vi "connectCommandPublish.vi"(8 "error in (no error)":errorcluster, 11 "MiddlewareSVThisComponent in":refnum<class "MiddlewareSVThisComponent.lvclass">) -> (0 "error out":errorcluster, 3 "MiddlewareSVThisComponent out":refnum<class "MiddlewareSVThisComponent.lvclass">)   [LabVIEW 2015, in "MiddlewareSVThisComponent.lvclass"]
uses:
  MiddlewareSVThisComponent.lvclass
  ComponentTemplateCore/ComponentModel/ComponentModel/Typedefs/CommunicationConfig.ctl
  ComponentTemplateCore/ComponentModel/ComponentModel/Typedefs/SVProcessConfig.ctl
  ComponentTemplateCore/ComponentModel/ComponentModelDT/ConfigurationFileReaderDT/ConfigurationFileReaderDT.lvclass
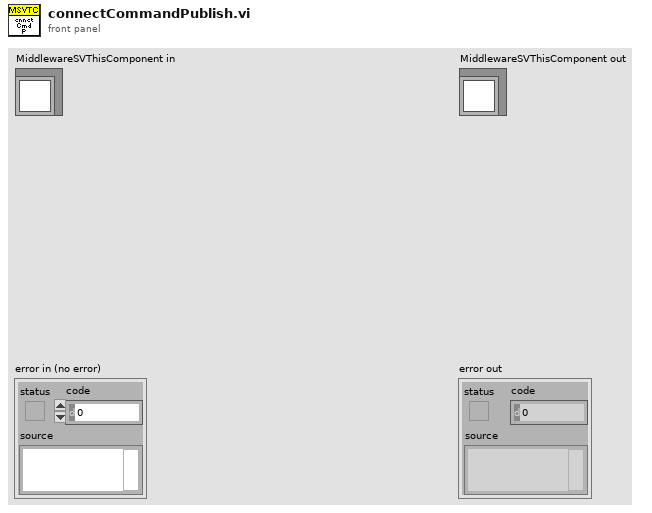
[diagram p1: front panel]
types:
  T1 = typedef "SVProcessConfig.ctl" = cluster{"subDataProcessPrototype":string, "pubDataProcessPrototype":string, "commandProcessPrototype":string, "commandSVName":string}
  T2 = typedef "CommunicationConfig.ctl" = cluster{"hostComputerAddress":string, "ComponentAcronym":string, "InstanceIdentifier":i32}
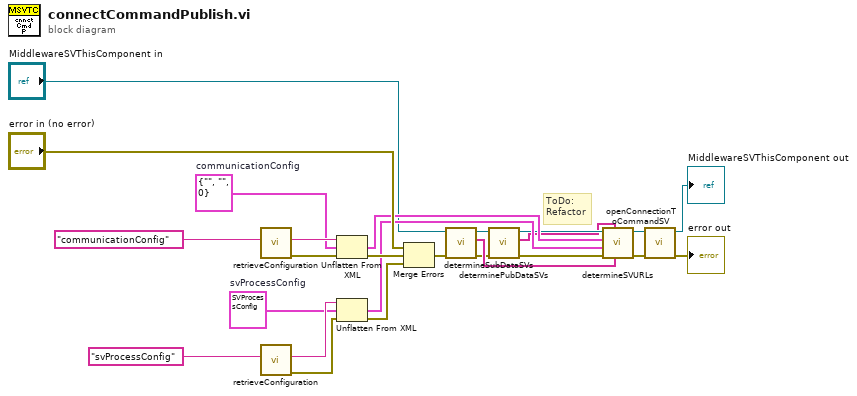
[diagram p0: block diagram]
diagram:
  w18 = T1 {"subDataProcessPrototype"="SubDataSV", "pubDataProcessPrototype"="PubDataSV", "commandProcessPrototype"="CommandSV", "commandSVName"="Command"}  # svProcessConfig
  w22 = T2 {"hostComputerAddress"="", "ComponentAcronym"="", "InstanceIdentifier"=0}  # communicationConfig
  # "ToDo:\nRefactor"
  n1 = call "retrieveConfiguration.vi"("dataName"="communicationConfig") -> ("error out"=w23:errorcluster, "dataValueFromFile"=w24:string)  [unwired: 8 in, 1 out]
  n2 = call "retrieveConfiguration.vi"("dataName"="svProcessConfig") -> ("error out"=w21:errorcluster, "dataValueFromFile"=w20:string)  [unwired: 8 in, 1 out]
  n3 = Unflatten From XML(xml string=w24, type=w22, error in (no error)=w23) -> (value=w9:T2, error out=w17:errorcluster)
  n4 = Unflatten From XML(xml string=w20, type=w18, error in (no error)=w21) -> (value=w10:T1, error out=w16:errorcluster)
  n5 = Merge Errors("error in (no error)", w17, w16) -> (w7:errorcluster)
  n6 = call "determineSubDataSVs.vi"("error in (no error)"=w7, "MiddlewareSVThisComponent in"="MiddlewareSVThisComponent in") -> ("error out"=w2:errorcluster, "svNames"=w6:string[], "MiddlewareSVThisComponent out"=w5:refnum<class "MiddlewareSVThisComponent.lvclass">)  [unwired: 7 in]
  n7 = call "determinePubDataSVs.vi"("error in (no error)"=w2, "MiddlewareSVThisComponent in"=w5) -> ("error out"=w1:errorcluster, "svNames"=w3:string[], "MiddlewareSVThisComponent out"=w4:refnum<class "MiddlewareSVThisComponent.lvclass">)  [unwired: 7 in]
  n8 = call-dynamic "determineSVURLs.vi"("subDataSVNames"=w6, "pubDataSVNames"=w3, "error in (no error)"=w1, "svProcessConfig"=w10, "communicationConfig"=w9, "MiddlewareSV in"=w4) -> ("error out"=w12:errorcluster, "MiddlewareSV out"=w14:refnum<class "MiddlewareSVThisComponent.lvclass">)  [unwired: 4 in]
  n9 = call-dynamic "openConnectionToCommandSV.vi"("error in (no error)"=w12, "MiddlewareSV in"=w14) -> ("error out"=→"error out":errorcluster, "MiddlewareSV out"=→"MiddlewareSVThisComponent out":refnum<class "MiddlewareSVThisComponent.lvclass">)  [unwired: 8 in]
